vi "Send Product.vi"(8 "error in (no error)":errorcluster, 9 "index":u16, 10 "Item Names":string[][](array[string]), 11 "Coca in":refnum<class "Coca.lvclass">) -> (0 "error out":errorcluster, 3 "Coca out":refnum<class "Coca.lvclass">)   [LabVIEW 2020, in "Coca.lvlib" / "Coca.lvclass"]
uses:
  Coca.lvclass
  C:/Program Files (x86)/National Instruments/LabVIEW 2020/vi.lib/ActorFramework/Actor/Actor.lvclass
  <vilib>/ActorFramework/Actor/Actor.lvclass/Actor.ctl
  Coca.lvclass/Coca.ctl
  UI Actor Messages/Actualiza MSG Msg/Actualiza MSG Msg.lvclass/Actualiza MSG Msg.ctl
  <vilib>/ActorFramework/Message Enqueuer/Message Enqueuer.lvclass/Message Enqueuer.ctl
  <vilib>/ActorFramework/Message Enqueuer/Enqueue.vi
  UI Actor Messages/Actualiza MSG Msg/Actualiza MSG Msg.lvclass
  C:/Program Files (x86)/National Instruments/LabVIEW 2020/vi.lib/ActorFramework/Message/Message.lvclass
  <vilib>/ActorFramework/Message Priority Queue/Priority Enqueue.vi
  <vilib>/ActorFramework/Actor/Actor.lvclass
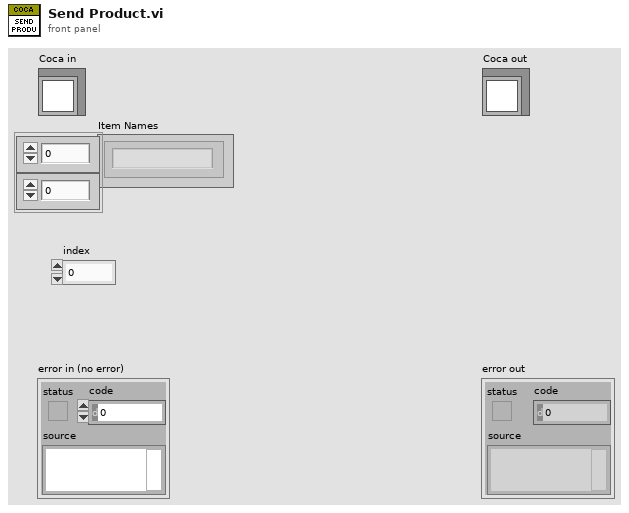
[diagram p1: front panel]
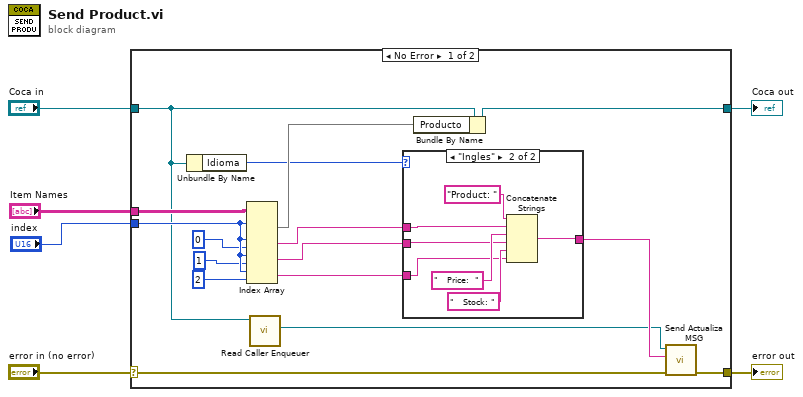
[diagram p0: block diagram]
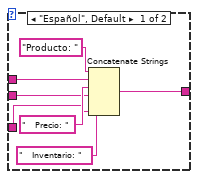
[diagram p2: hidden frame]
diagram:
  n1 = case shown="No Error" "error in (no error)" {
    selector: "error in (no error)" -> [w20 w38]
    tunnel: [w19 w38] -> w5
    tunnel: [w11 w37] -> w3
    tunnel: "Coca in" -> [w8 w37]
    tunnel: "Item Names" -> [w22 _]
    tunnel: "index" -> [w17 _]
    frame No Error {
      n2 = Unbundle By Name(w8) -> ("Idioma"=w7:enum16{"Español", "Ingles"})
      n3 = Index Array(array=w22, index (row) #1=w17, index (row) #2=w17, index (col) #2=0 ("disabled index (col)"), index (row) #3=w17, index (col) #3=1 ("disabled index (col)"), index (row) #4=w17, index (col) #4=2 ("disabled index (col)")) -> (element #1=w10:string[], element #2=w12:string, element #3=w13:string, element #4=w14:string)  [unwired: 1 in]
      n4 = call <vilib>:"Read Caller Enqueuer.vi"("Actor"=w8) -> ("Caller Enqueuer"=w18:refnum<class "Message Enqueuer.lvclass">)  [unwired: 10 in]
      n5 = case shown="\"Ingles\"" w7 {
        tunnel: [w26 w30] -> w21
        tunnel: w14 -> [w25 w31]
        tunnel: w13 -> [w24 w33]
        tunnel: w12 -> [w23 w34]
        frame "Español", Default {
          n6 = Concatenate Strings("Producto: " ("string"), w23, "   Precio: " ("string"), w24, "   Inventario: " ("string"), w25) -> (w26:string)
        }
        frame "Ingles" {
          n7 = Concatenate Strings("Product: " ("string"), w34, "   Price:  " ("string"), w33, "   Stock: " ("string"), w31) -> (w30:string)
        }
      }
      n8 = Bundle By Name(cluster=w8, "Producto"=w10) -> (w11:refnum<class "Coca.lvclass">)
      n9 = call "Send Actualiza MSG.vi"("error in (no error)"=w20, "MSG"=w21, "Message Enqueuer"=w18) -> ("error out"=w19:errorcluster)  [unwired: 7 in, 1 out]
    }
    frame Error {
    }
  }
  "error out" <- w5
  "Coca out" <- w3
